vi "停止判断1.vi"(6 "重置？":bool, 7 "反转？":bool, 8 "error in (no error)":errorcluster caption="错误输入（无错误）", 9 "停止判断条件1":T1, 10 "传感器数据":dbl[](array[numeric]), 11 "Message Queue":refnum<queue> caption="消息队列") -> (0 "error out":errorcluster caption="错误输出", 3 "Message Queue 2":refnum<queue> caption="消息队列")   [LabVIEW 2015, in "Action.lvlib"]
uses:
  Action.lvlib
  support/Message Queue/Message Cluster.ctl
  support/Message Queue/Enqueue Message (Single).vi
  support/Message Queue/Message Queue.lvlib
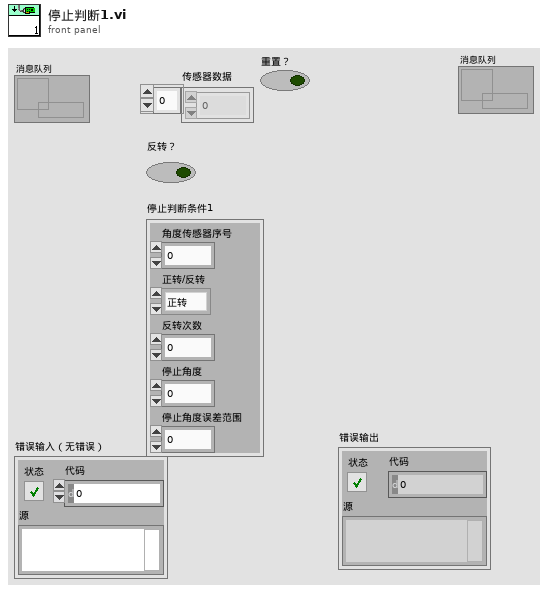
[diagram p1: front panel]
types:
  T1 = typedef "Action.lvlib/停止判断条件1.ctl" = cluster{"角度传感器序号":i32, "正转/反转":enum16{"正转", "反转"}, "反转次数":i32, "停止角度":dbl, "停止角度误差范围":dbl}
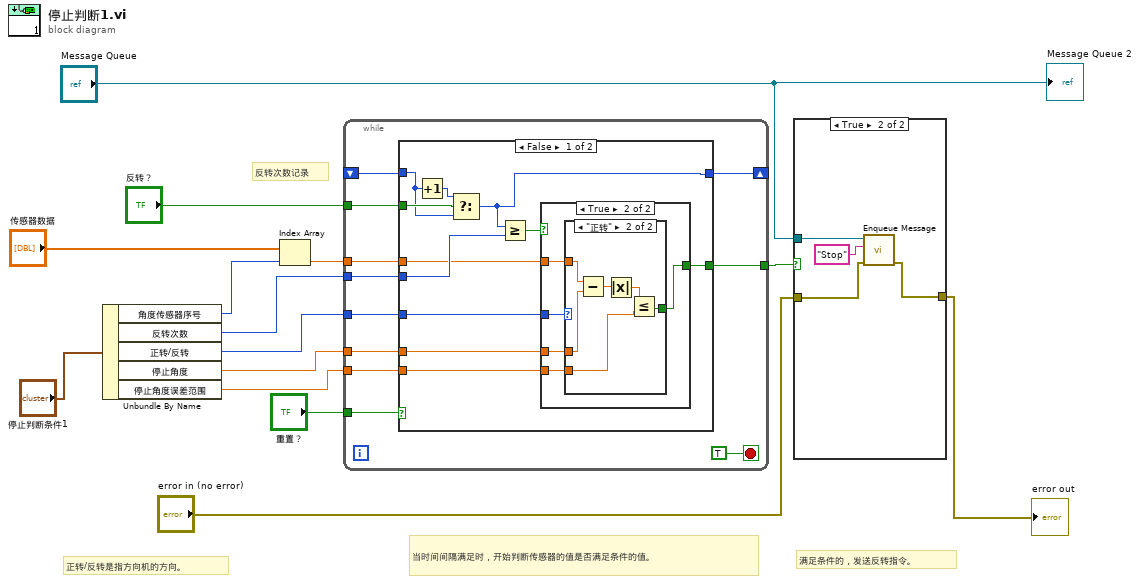
[diagram p0: block diagram]
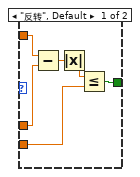
[diagram p4: hidden frame]
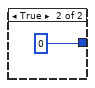
[diagram p5: hidden frame]
diagram:
  # "正转/反转是指方向机的方向。"
  # "满足条件的，发送反转指令。"
  # "当时间间隔满足时，开始判断传感器的值是否满足条件的值。"
  # "反转次数记录"
  n1 = Unbundle By Name("停止判断条件1") -> ("角度传感器序号"=w4:i32, "反转次数"=w12:i32, "正转/反转"=w3:enum16{"正转", "反转"}, "停止角度"=w10:dbl, "停止角度误差范围"=w9:dbl)
  n2 = Index Array(array="传感器数据", index=w4) -> (element=w11:dbl)
  n3 = while {
    tunnel: w12 -> [w25]
    tunnel: w11 -> [w24]
    tunnel: w10 -> [w23]
    shift-right: [w22] -> _
    shift-left: _ -> [w16]
    tunnel: w9 -> [w21]
    tunnel: [w20] -> w8
    tunnel: "反转？" -> [w18]
    tunnel: w3 -> [w17]
    tunnel: "重置？" -> [w15]
    stop <- TRUE stop-if-true
    n4 = case shown="False" w15 {
      tunnel: w25 -> [w32 _]
      tunnel: w24 -> [w30 _]
      tunnel: w23 -> [w28 _]
      tunnel: [w33 0] -> w22
      tunnel: w16 -> [w34 _]
      tunnel: w21 -> [w27 _]
      tunnel: [w26 _] -> w20
      tunnel: w18 -> [w36 _]
      tunnel: w17 -> [w29 _]
      frame False {
        n5 = Increment(x=w34) -> (x+1=w35:i32)
        n6 = Select(t=w35, s=w36, f=w34) -> (s? t:f=w33:i32)
        n7 = Greater Or Equal?(x=w33, y=w32) -> (x >= y?=w31:bool)
        n8 = case shown="True" w31 {
          tunnel: w30 -> [_ w41]
          tunnel: w29 -> [_ w37]
          tunnel: w28 -> [_ w40]
          tunnel: w27 -> [_ w39]
          tunnel: [_ w38] -> w26
          frame False {
          }
          frame True {
            n9 = case shown="\"正转\"" w37 {
              tunnel: w41 -> [w47 w53]
              tunnel: w40 -> [w46 w52]
              tunnel: w39 -> [w45 w50]
              tunnel: [w44 w48] -> w38
              frame "反转", Default {
                n10 = Subtract(x=w47, y=w46) -> (x-y=w43:dbl)
                n11 = Absolute Value(x=w43) -> (abs(x)=w42:dbl)
                n12 = Less Or Equal?(x=w42, y=w45) -> (x <= y?=w44:bool)
              }
              frame "正转" {
                n13 = Subtract(x=w53, y=w52) -> (x-y=w51:dbl)
                n14 = Absolute Value(x=w51) -> (abs(x)=w49:dbl)
                n15 = Less Or Equal?(x=w49, y=w50) -> (x <= y?=w48:bool)
              }
            }
          }
        }
      }
      frame True {
      }
    }
  }
  n16 = case shown="True" w8 {
    tunnel: "Message Queue" -> [_ w59]
    tunnel: "error in (no error)" -> [w55 w58]
    tunnel: [w55 w57] -> w6
    frame False {
    }
    frame True {
      n17 = call-poly "Enqueue Message.vi"("error in (no error)"=w58, "Message"="Stop", "Message Queue"=w59) -> ("error out"=w57:errorcluster)  [unwired: 7 in, 1 out]
    }
  }
  "error out" <- w6
  "Message Queue 2" <- "Message Queue"
